vi "Logger.Stats.Find.vi"(8 "error in (no error)":errorcluster) -> (0 "error out":errorcluster, 2 "#loaded entries":i32)   [LabVIEW 2016]
uses:
  Global/ApplicationGlobal.vi
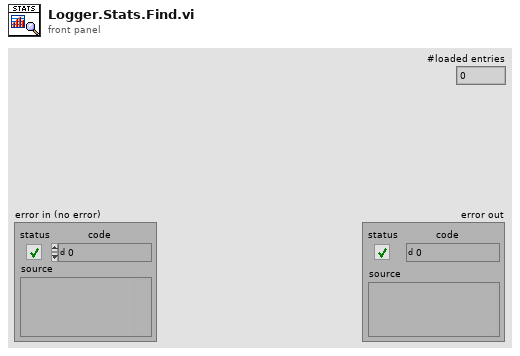
[diagram p1: front panel]
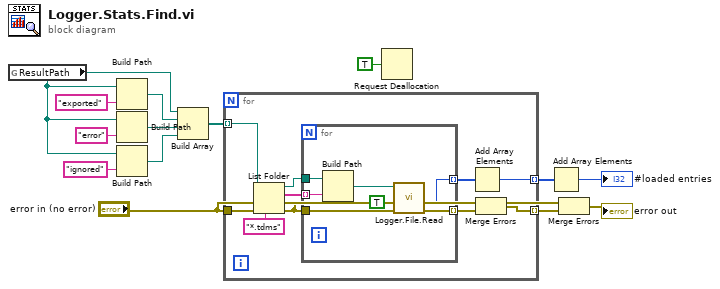
[diagram p0: block diagram]
diagram:
  n1 = global read "ApplicationGlobal.vi" "ResultPath"() -> (w6:path)
  n2 = Build Path(base path=w6, name or relative path="exported") -> (appended path=w10:path)
  n3 = Build Path(base path=w6, name or relative path="error") -> (appended path=w7:path)
  n4 = Build Path(base path=w6, name or relative path="ignored") -> (appended path=w9:path)
  n5 = Build Array(w6, w10, w7, w9) -> (w8:path[])
  n6 = for {
    tunnel: w8 -> [w23] mode=indexing
    tunnel: "error in (no error)" -> [w24]
    tunnel: [w18] -> w3 mode=indexing
    tunnel: [w16] -> w2 mode=indexing
    n7 = List Folder(path=w23, pattern="*.tdms", error in=w24) -> (path out=w21:path, filenames=w22:string[], error out=w15:errorcluster)  [unwired: 1 in, 1 out]
    n8 = for {
      tunnel: w22 -> [w31] mode=indexing
      tunnel: w21 -> [w30]
      tunnel: w15 -> [w29]
      tunnel: [w26] -> w19 mode=indexing
      tunnel: [w25] -> w17 mode=indexing
      n9 = Build Path(base path=w30, name or relative path=w31) -> (appended path=w28:path)
      n10 = call "Logger.File.Read.vi"("error in (no error)"=w29, "Update Stats (F)"=TRUE, "file path"=w28) -> ("error out"=w26:errorcluster, "Stats elements"=w25:i32)  [unwired: 5 in, 2 out]
    }
    n11 = Add Array Elements(numeric array=w17) -> (sum=w16:i32)
    n12 = Merge Errors(w15, w19) -> (w18:errorcluster)
  }
  n13 = Request Deallocation(TRUE ("flag")) -> ()
  n14 = Add Array Elements(numeric array=w2) -> (sum=→"#loaded entries":i32)
  n15 = Merge Errors("error in (no error)", w3) -> (→"error out":errorcluster)
